vi "templateboard2.vi"(9 "board array":i16[][](array[numeric])) -> (1 "Picture":picture)   [LabVIEW 2018]
panel:
  in  "Block Size (20)":u32=20
  in  "color array":u32[](array[colorbox])=[0, 15790080, 8388608, 8421376, 128, 32896, 8388736, 32896]
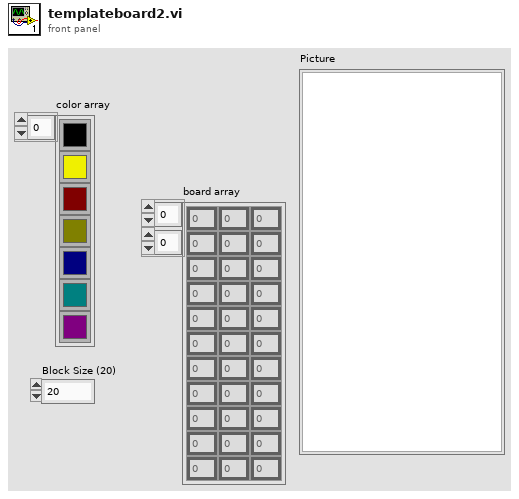
[diagram p1: front panel]
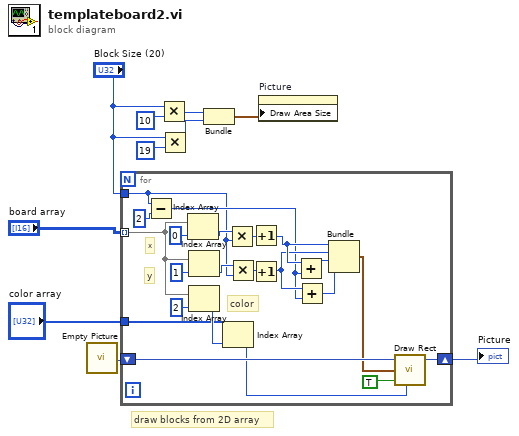
[diagram p0: block diagram]
diagram:
  # "draw blocks from 2D array"
  n1 = call "Empty Picture"() -> ("empty picture"=w3:picture)
  n2 = for {
    shift-right: [w19] -> w2
    shift-left: w3 -> [w20]
    tunnel: "board array" -> [w29] mode=indexing
    tunnel: "Block Size (20)" -> [w11]
    tunnel: "color array" -> [w27]
    # "y"
    # "x"
    # "color"
    n3 = Subtract(x=w11, y=u32 2) -> (x-y=w23:u32)
    n4 = Index Array(array=w29, index=0) -> (element=w15:i16)
    n5 = Index Array(array=w29, index=1) -> (element=w14:i16)
    n6 = Index Array(array=w29, index=2) -> (element=w28:i16)
    n7 = Index Array(array=w27, index=w28) -> (element=w16:u32)
    n8 = Multiply(x=w15, y=w11) -> (x*y=w12:u32)
    n9 = Multiply(x=w14, y=w11) -> (x*y=w13:u32)
    n10 = Increment(x=w12) -> (x+1=w25:u32)
    n11 = Increment(x=w13) -> (x+1=w24:u32)
    n12 = Add(x=w25, y=w23) -> (x+y=w22:u32)
    n13 = Add(x=w24, y=w23) -> (x+y=w21:u32)
    n14 = Bundle(w25, w24, w22, w21) -> (w18:cluster{u32, u32, u32, u32})  [unwired: 1 in]
    n15 = call <vilib>:"Draw Rect.vi"("picture"=w20, "rect"=w18, "fill?(F)"=TRUE, "color(black)"=w16) -> ("new picture"=w19:picture)  [unwired: 5 in]
  }
  "Picture" <- w2
  n16 = Multiply(x="Block Size (20)", y=u32 10) -> (x*y=w5:u32)
  n17 = Multiply(x="Block Size (20)", y=u32 19) -> (x*y=w4:u32)
  n18 = Bundle(w5, w4) -> (w8:cluster{u32, u32})  [unwired: 1 in]
  n19 = property on="Picture" class="Pict"("Draw Area Size"=w8) -> ()  [unwired: 2 in, 2 out]
